vi "SetPrinterBusy_Status_GIS Printer.vi"(8 "error in (no error)":errorcluster, 10 "Printer Busy?":bool, 11 "GIS Printer In":refnum<class "GIS Printer.lvclass">) -> (0 "error out":errorcluster, 3 "GIS Printer Out":refnum<class "GIS Printer.lvclass">)   [LabVIEW 2022 SP3, in "GIS Printer.lvclass"]
uses:
  GIS Printer.lvclass
  GIS Printer.lvclass/GIS Printer.ctl
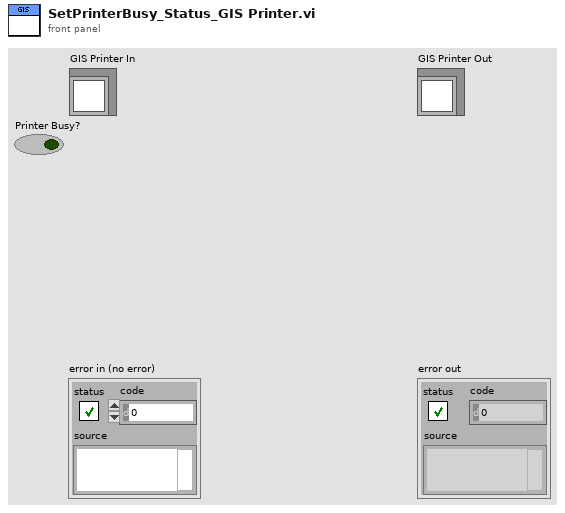
[diagram p1: front panel]
types:
  T1 = typedef "GIS Printer.lvclass/Private Data.ctl" = cluster{"UserEvents":T2, "All Dependencies":cluster{"Class References":refnum<class>[], "Class Names":string[]}, "PrinterConiguration":T3, "Status":T4, "GISHeadStatus":T5[], "HeadStatus":T6}
  T2 = typedef "GIS Printer.lvclass/UserEvents.ctl" = cluster{"API Incoming Event":refnum<user-event>, "API Executed Event":refnum<user-event>, "API Return Event":refnum<user-event>, "Status Changed Event":refnum<user-event>, "Abort":refnum<user-event>, "stop process":refnum<user-event>, "GISPollStatus":refnum<user-event>, "GISHeadStatus":refnum<user-event>}
  T3 = typedef "GIS Printer.lvclass/PrinterConfiguration--Cluster.ctl" = cluster{"IPAddress":string, "Move Stage on RTP Command?":bool, "Stage Move Position":string, "PH1-Prime Path":path, "PH2-Prime Path":path, "PH3-Prime Path":path, "PH4-Prime Path":path, "PH5-Prime Path":path, "PH6-Prime Path":path, "PrintScriptsFolder":path, "PurgeScriptsFolder":path, "StageScriptsFolder":path, "PH1-HeatOn Path":path, "PH2-HeatOn Path":path, "PH3-HeatOn Path":path, "PH4-HeatOn Path":path, "PH5-HeatOn Path":path, "PH6-HeatOn Path":path, "PH1-HeatOff Path":path, "PH2-HeatOff Path":path, "PH3-HeatOff Path":path, "PH4-HeatOff Path":path, "PH5-HeatOff Path":path, "PH6-HeatOff Path":path}
  T4 = typedef "GIS Printer.lvclass/Status Cluster.ctl" = cluster{"Command Status":variant, "TCP Commands & Responses":string[][], "Printer Busy?":bool}
  T5 = typedef "GIS Status--Cluster.ctl" = cluster{"HeadEnabled":bool, "SpitEnabled":bool, "HeaterEnabled":bool, "TargetTemperature":dbl, "CurrentTemperature":dbl}
  T6 = typedef "HeadEnableStatus--cluster.ctl" = cluster{"PH1_Enable":bool, "PH2_Enable":bool, "PH3_Enable":bool, "PH4_Enable":bool, "PH5_Enable":bool, "PH6_Enable":bool}
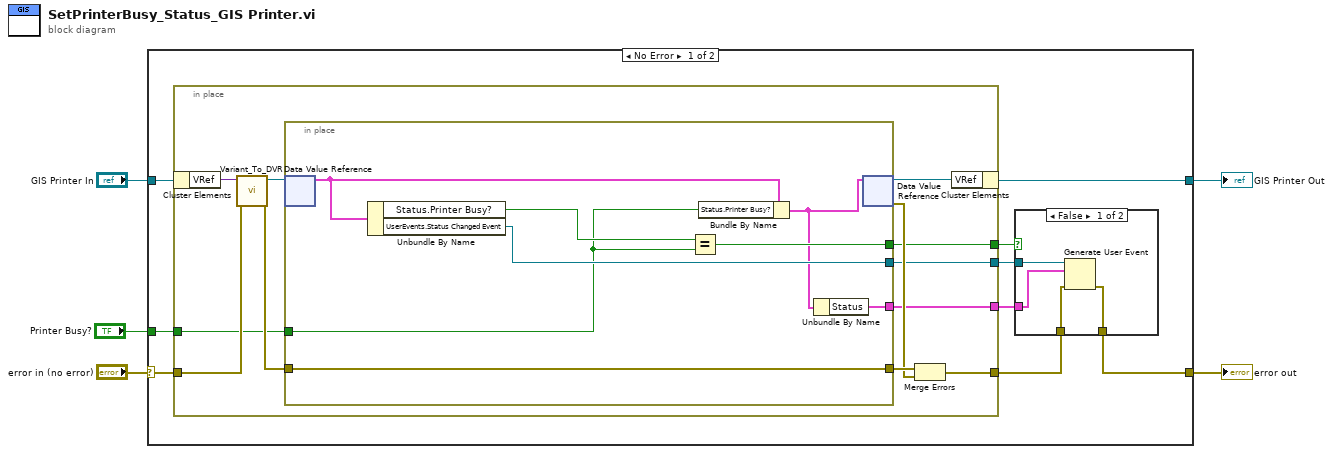
[diagram p0: block diagram]
diagram:
  n1 = case shown="No Error" "error in (no error)" {
    selector: "error in (no error)" -> [w12 w41]
    tunnel: [w10 w41] -> w4
    tunnel: [w14 w40] -> w2
    tunnel: "GIS Printer In" -> [w13 w40]
    tunnel: "Printer Busy?" -> [w8 _]
    frame No Error {
      n2 = in-place {
        in-place-border: w12 -> [w29]
        in-place-border: [w25] -> w11
        in-place-border: [w23] -> w9
        in-place-border: w8 -> [w22]
        in-place-border: [w21] -> w7
        in-place-border: [w20] -> w6
        n3 = in-place-cluster #1(w13) -> ("VRef"=w31:variant)
        n4 = call "Variant_To_DVR.vi"("error in (no error)"=w29, "Variant"=w31) -> ("error out"=w28:errorcluster, "DVR"=w30:refnum<data-value>)  [unwired: 8 in]
        n5 = in-place {
          in-place-border: w28 -> [w39]
          in-place-border: [w39] -> w27
          in-place-border: [w37] -> w23
          in-place-border: w22 -> [w35]
          in-place-border: [w34] -> w21
          in-place-border: [w32] -> w20
          n6 = in-place-dvr #2(w30) -> (w38:T1)  [unwired: 1 out]
          n7 = Unbundle By Name(w38) -> ("Status.Printer Busy?"=w36:bool, "UserEvents.Status Changed Event"=w37:refnum<user-event>)
          n8 = Equal?(x=w36, y=w35) -> (x = y?=w34:bool)
          n9 = Bundle By Name(cluster=w38, "Status.Printer Busy?"=w35) -> (w33:T1)
          n10 = Unbundle By Name(w33) -> ("Status"=w32:T4)
          n11 = in-place-dvr #2(w33) -> (w24:refnum<data-value>, w26:errorcluster)
        }
        n12 = Merge Errors(w27, w26) -> (w25:errorcluster)
        n13 = in-place-cluster #1("VRef"=w24) -> (w14:refnum<class "GIS Printer.lvclass">)
      }
      n14 = case shown="False" w7 {
        tunnel: w11 -> [w18 w19]
        tunnel: [w17 w19] -> w10
        tunnel: w9 -> [w16 _]
        tunnel: w6 -> [w15 _]
        frame False {
          n15 = Generate User Event(user event=w16, event data cluster=w15, error in=w18) -> (error out=w17:errorcluster)  [unwired: 1 in, 1 out]
        }
        frame True {
        }
      }
    }
    frame Error {
    }
  }
  "error out" <- w4
  "GIS Printer Out" <- w2
